vi "x4xx usrp aurora streaming.vi"() -> ()   [LabVIEW 2023]
panel:
  in  "Radio1 Configuration":T1={"Ch1 Rx Frequency"=2000000000.0, "Ch1 Tx Frequency"=2000000000.0, "Ch1 Rx Gain"=0.0, "Ch1 Tx Gain"=0.0} {"Ch1 Tx Frequency" format="%#_6p"; "Ch1 Rx Frequency" format="%#_6p"}
  in  "Radio0 Configuration":T2={"Ch0 Rx Frequency"=2000000000.0, "Ch0 Tx Frequency"=2000000000.0, "Ch0 Rx Gain"=0.0, "Ch0 Tx Gain"=0.0} {"Ch0 Tx Frequency" format="%#_6p"; "Ch0 Rx Frequency" format="%#_6p"}
  in  "Channels":enum16{"0", "1", "0,1"}(ring)
  out "USRP Aurora Errors":T3(array[cluster])
  out "USRP Aurora Status":T4(array[cluster])
  in  "stop acquisition":bool
  in  "start acquisition":bool
  in  "disable generation":bool
  in  "enable generation":bool
  in  "USRP arguments":string="addr=192.167.11.2,master_clock_rate=125e6"
  out "on":bool caption="Connected"
  in  "stop":bool
  out "error out":errorcluster
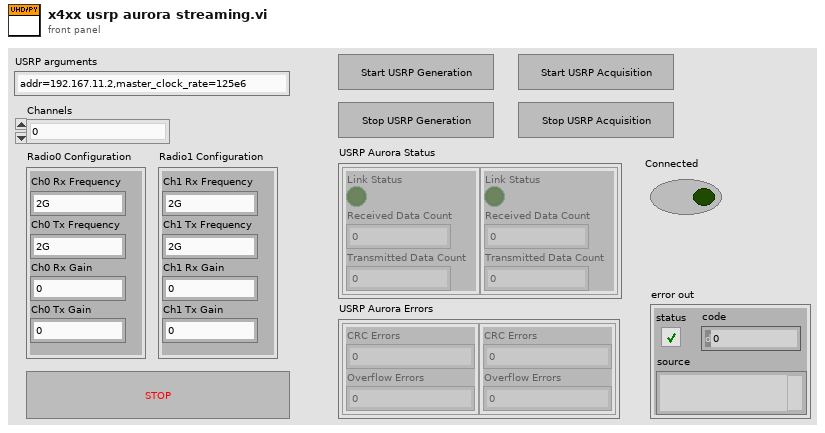
[diagram p1: front panel]
types:
  T1 = cluster{"Ch1 Rx Frequency":dbl, "Ch1 Tx Frequency":dbl, "Ch1 Rx Gain":dbl, "Ch1 Tx Gain":dbl}
  T2 = cluster{"Ch0 Rx Frequency":dbl, "Ch0 Tx Frequency":dbl, "Ch0 Rx Gain":dbl, "Ch0 Tx Gain":dbl}
  T3 = cluster{"CRC Errors":i32, "Overflow Errors":i32}[]
  T4 = cluster{"Link Status":bool, "Received Data Count":i32, "Transmitted Data Count":i32}[]
  T5 = cluster{"python path":path, "session out":refnum<k35>, "uhd graph":refnum<k38>}
  T6 = cluster{"python path":path, "session out ":refnum<k35>, "uhd graph":refnum<k38>}
  T7 = cluster{"link_status":bool, "rx_count":i32, "tx_count":i32}[]
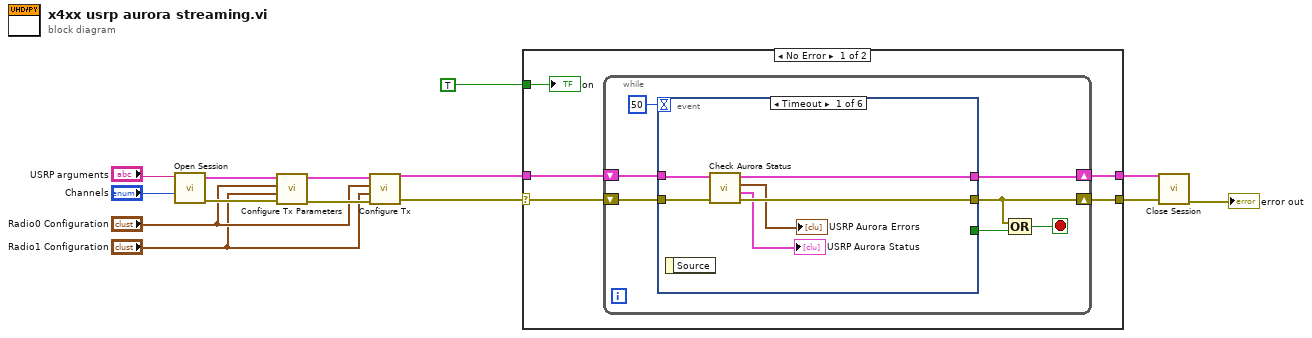
[diagram p0: block diagram]
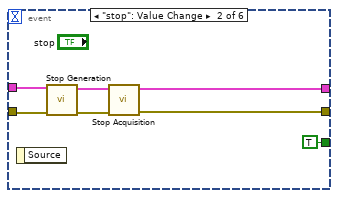
[diagram p2: hidden frame]
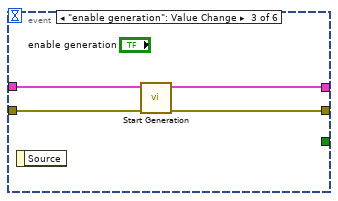
[diagram p3: hidden frame]
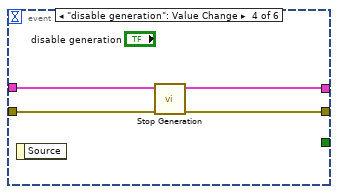
[diagram p4: hidden frame]
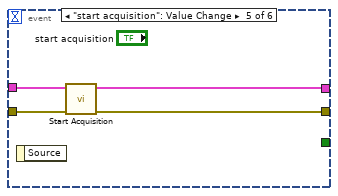
[diagram p5: hidden frame]
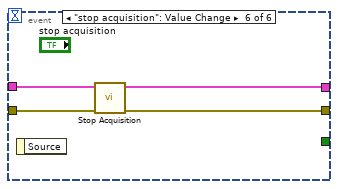
[diagram p6: hidden frame]
diagram:
  n1 = call "Open Session.vi"("Channels"="Channels", "x4xx argument"="USRP arguments") -> ("error out"=w12:errorcluster, "Session Out"=w6:T5)  [unwired: 8 in]
  n2 = call "Configure Tx Parameters.vi"("error in"=w12, "Radio1 Configuration"="Radio1 Configuration", "Radio0 Configuration"="Radio0 Configuration", "session In"=w6) -> ("error out"=w11:errorcluster, "session out"=w5:T6)  [unwired: 6 in]
  n3 = call "Configure Tx.vi"("error in"=w11, "Radio1 Configuration"="Radio1 Configuration", "Radio0 Configuration"="Radio0 Configuration", "session in"=w5) -> ("error out"=w9:errorcluster, "session out"=w10:T5)  [unwired: 6 in]
  n4 = case shown="No Error" w9 {
    selector: w9 -> [w17 w57]
    tunnel: [w19 w57] -> w7
    tunnel: TRUE -> [w18 _]
    tunnel: w10 -> [w16 w56]
    tunnel: [w15 w56] -> w4
    frame No Error {
      n5 = while {
        shift-right: [w23] -> w19
        shift-left: w17 -> [w26]
        shift-right: [w20] -> w15
        shift-left: w16 -> [w21]
        stop <- w24 stop-if-true
        n6 = event shown="[0] Timeout" {
          selector: _ -> [_ _ _ _ _ _]
          dyn-events: _ -> [_ _ _ _ _ _]
          timeout: 50 -> [_ _ _ _ _ _]
          tunnel: [w32 w33 w42 w46 w50 w54] -> w23
          tunnel: w26 -> [w31 w37 w43 w47 w51 w55]
          tunnel: [_ TRUE _ _ _ _] -> w25
          tunnel: w21 -> [w30 w38 w41 w45 w49 w53]
          tunnel: [w29 w34 w40 w44 w48 w52] -> w20
          event Timeout {
            n7 = event-data() -> ()  [unwired: 1 in, 1 out]
            n8 = call "Check Aurora Status.vi"("error in"=w31, "session In"=w30) -> ("error out"=w32:errorcluster, "USRP Aurora Status"=→"USRP Aurora Status":T7, "USRP Aurora Errors"=→"USRP Aurora Errors":cluster{"crc_errors":i32, "overflows":i32}[], "session out"=w29:T5)  [unwired: 6 in]
          }
          event "stop": Value Change {
            n9 = event-data() -> ()  [unwired: 1 in, 1 out]
            n10 = call "Stop Generation.vi"("error in"=w37, "session In"=w38) -> ("error out"=w35:errorcluster, "session out"=w36:T6)  [unwired: 8 in]
            n11 = call "Stop Acquisition.vi"("error in"=w35, "session In"=w36) -> ("error out"=w33:errorcluster, "session out"=w34:T6)  [unwired: 8 in]
          }
          event "enable generation": Value Change {
            n12 = event-data() -> ()  [unwired: 1 in, 1 out]
            n13 = call "Start Generation.vi"("error in"=w43, "session In"=w41) -> ("error out"=w42:errorcluster, "session out"=w40:T5)  [unwired: 8 in]
          }
          event "disable generation": Value Change {
            n14 = event-data() -> ()  [unwired: 1 in, 1 out]
            n15 = call "Stop Generation.vi"("error in"=w47, "session In"=w45) -> ("error out"=w46:errorcluster, "session out"=w44:T6)  [unwired: 8 in]
          }
          event "start acquisition": Value Change {
            n16 = event-data() -> ()  [unwired: 1 in, 1 out]
            n17 = call "Start Acquisition.vi"("error in (no error)"=w51, "session In"=w49) -> ("error out"=w50:errorcluster, "session out"=w48:T6)  [unwired: 8 in]
          }
          event "stop acquisition": Value Change {
            n18 = event-data() -> ()  [unwired: 1 in, 1 out]
            n19 = call "Stop Acquisition.vi"("error in"=w55, "session In"=w53) -> ("error out"=w54:errorcluster, "session out"=w52:T6)  [unwired: 8 in]
          }
        }
        n20 = Compound Arithmetic op=OR(w23, w25) -> (w24:bool)
      }
      "on" <- w18
    }
    frame Error {
    }
  }
  n21 = call "Close Session.vi"("error in"=w7, "session In"=w4) -> ("error out"=→"error out":errorcluster)  [unwired: 9 in]
